vi "Many N Field Set Com.vi"() -> (0 "Command text":string[][](array[string]))   [LabVIEW 2024]
uses:
  Field Set.ctl
panel:
  in  "Slew Rate (T/min)":dbl
  in  "Initial Field":dbl
  in  "Final Field":dbl
  in  "Number of Interval":dbl
  in  "Generate":bool
  in  "cancel":bool
  in  "next":bool
  in  "SetFieldCluster":T1={"rate"=0.0, "set point"=1.0, "extra wait"=0, "wait option"=1} {"wait option" items=["Do not wait, just move on", "Wait until it reaches the set point."]; "extra wait" min=0; "set point" format="%.5f"; "rate" format="%.5f"}
  in  "wait after each field (sec)":i32
  out "loop array":dbl[][](array[numeric])
  in  "Array":dbl[][](array[numeric]) format="%#_4e"
  # "Field Set (Multiple Input Generator)"
  # "generates multiple field set values for the sequence, see belolw.  If you like it click \"Good, use this!\". You can also modify the values directly from the following array."
  # "Field (T)"
  # "Set Field Command"
  # "T"
  # "at"
  # "T/min"
  # "1. Sweep field to"
  # "2. AND wait extra"
  # "seconds"
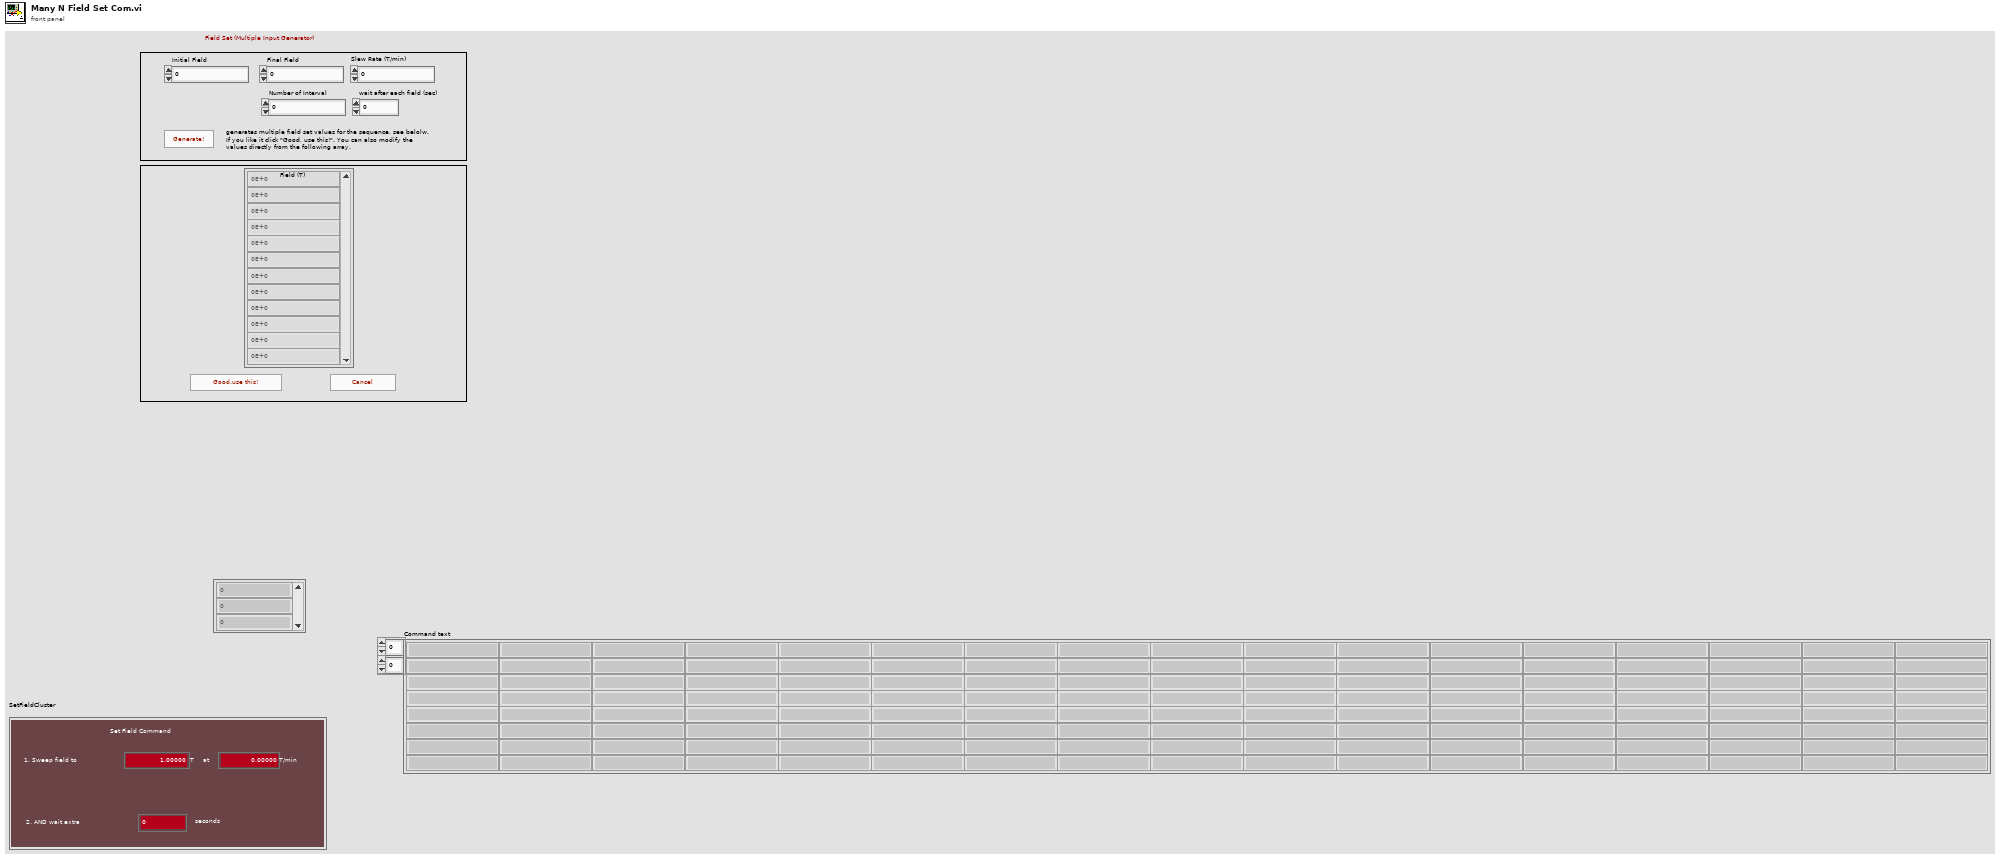
[diagram p1: front panel]
types:
  T1 = typedef "Field Set.ctl" = cluster{"rate":dbl, "set point":dbl, "extra wait":i32, "wait option":u16}
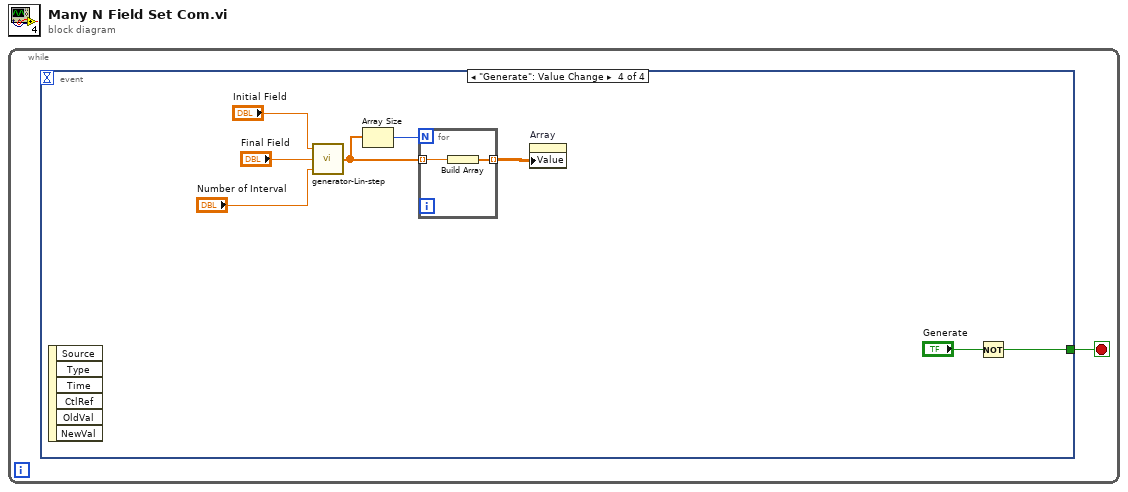
[diagram p0: block diagram]
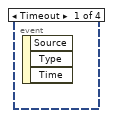
[diagram p2: hidden frame]
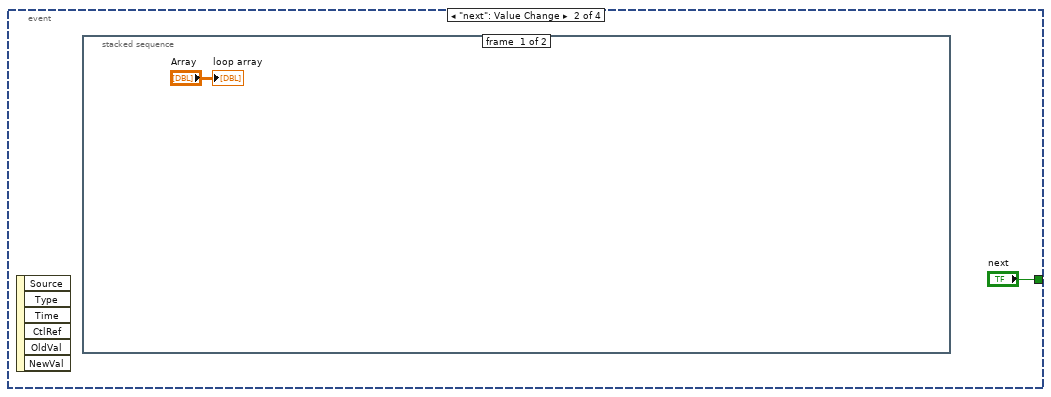
[diagram p3: hidden frame]
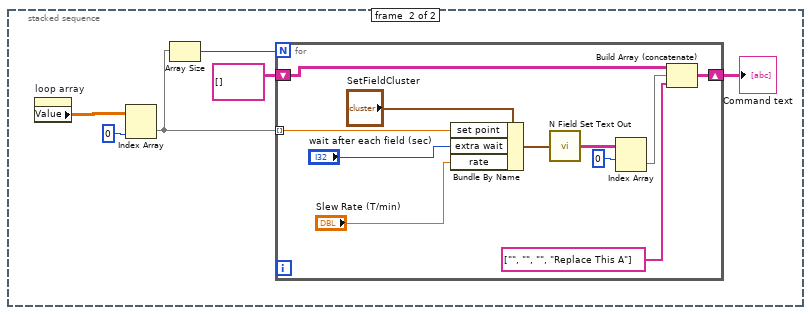
[diagram p4: hidden frame]
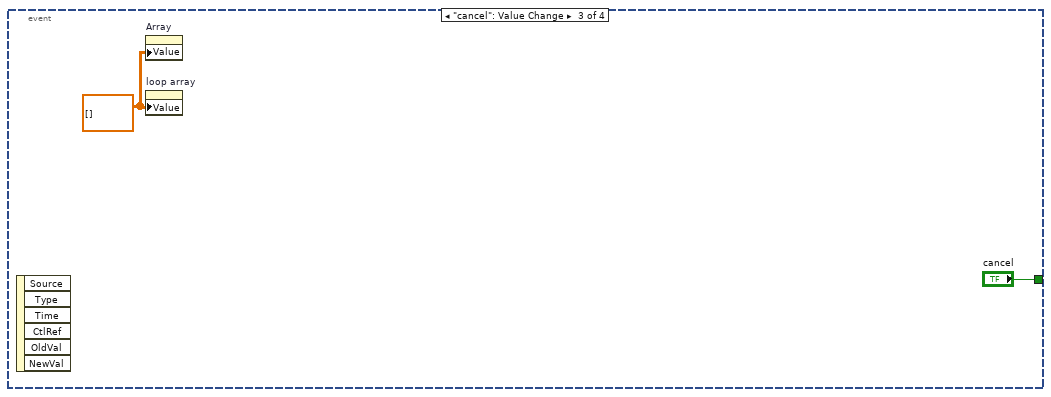
[diagram p5: hidden frame]
diagram:
  n1 = while {
    stop <- w1 stop-if-true
    n2 = event shown="[3] \"Generate\": Value Change" {
      selector: _ -> [_ _ _ _]
      dyn-events: _ -> [_ _ _ _]
      timeout: _ -> [_ _ _ _]
      tunnel: [_ "next" "cancel" w25] -> w1
      event Timeout {
        n3 = event-data() -> ()  [unwired: 1 in, 3 out]
      }
      event "next": Value Change {
        n4 = event-data() -> ()  [unwired: 1 in, 6 out]
        n5 = stacked-sequence {
          frame #0 {
            "loop array" <- "Array"
          }
          frame #1 {
            n6 = property on="loop array" class="Arr (strict)"() -> ("Value"=w8:dbl[][])  [unwired: 2 in, 2 out]
            n7 = Index Array(array=w8, index (col)=0 ("disabled index (col)")) -> (element=w7:dbl[])  [unwired: 1 in]
            n8 = Array Size(array=w7) -> (size(s)=w6:i32)
            n9 = for {
              N: w6 -> [_]
              tunnel: w7 -> [w12] mode=indexing
              shift-right: [w14] -> w5
              shift-left: string[][] [] -> [w13]
              n10 = Bundle By Name(cluster="SetFieldCluster", "set point"=w12, "extra wait"="wait after each field (sec)", "rate"="Slew Rate (T/min)") -> (w11:T1)
              n11 = call "N Field Set Text Out.vi"("SetFieldCluster"=w11) -> ("Command text"=w18:string[][])
              n12 = Index Array(array=w18, index (row)=0) -> (element=w16:string[])  [unwired: 1 in]
              n13 = Build Array (concatenate)(w13, w16, string[] ["", "", "", "Replace This A"]) -> (w14:string[][])
            }
            "Command text" <- w5
          }
        }
      }
      event "cancel": Value Change {
        w21 = dbl[][] [] ("Array")
        n14 = event-data() -> ()  [unwired: 1 in, 6 out]
        n15 = property on="Array" class="Arr (strict)"("Value"=w21) -> ()  [unwired: 2 in, 2 out]
        n16 = property on="loop array" class="Arr (strict)"("Value"=w21) -> ()  [unwired: 2 in, 2 out]
      }
      event "Generate": Value Change {
        n17 = event-data() -> ()  [unwired: 1 in, 6 out]
        n18 = call "generator-Lin-step.vi"("step"="Number of Interval", "end"="Final Field", "start"="Initial Field") -> ("Array"=w24:dbl[])
        n19 = Array Size(array=w24) -> (size(s)=w26:i32)
        n20 = for {
          N: w26 -> [_]
          tunnel: w24 -> [w32] mode=indexing
          tunnel: [w31] -> w23 mode=indexing
          n21 = Build Array(w32) -> (w31:dbl[])
        }
        n22 = property on="Array" class="Arr (strict)"("Value"=w23) -> ()  [unwired: 2 in, 2 out]
        n23 = Not(x="Generate") -> (.not. x?=w25:bool)
      }
    }
  }
